vi "Status_Error_Messages.vi"() -> ()   [LabVIEW 2012]
panel:
  in  "Status/Error messages":string
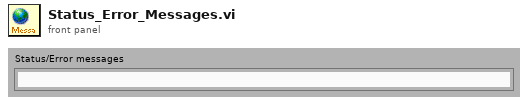
[diagram p1: front panel]
diagram:
